vi "worksheet filter column2 lv.vi"(4 "and_or":u8, 6 "lxw_filter_rule 2":T1 {"criteria" items=["LXW_FILTER_CRITERIA_NONE", "LXW_FILTER_CRITERIA_EQUAL_TO", "LXW_FILTER_CRITERIA_NOT_EQUAL_TO", "LXW_FILTER_CRITERIA_GREATER_THAN", "LXW_FILTER_CRITERIA_LESS_THAN", "LXW_FILTER_CRITERIA_GREATER_THAN_OR_EQUAL_TO", "LXW_FILTER_CRITERIA_LESS_THAN_OR_EQUAL_TO", "LXW_FILTER_CRITERIA_BLANKS", "LXW_FILTER_CRITERIA_NON_BLANKS"]}, 8 "error in (no error)":errorcluster, 9 "lxw_filter_rule":T1 {"criteria" items=["LXW_FILTER_CRITERIA_NONE", "LXW_FILTER_CRITERIA_EQUAL_TO", "LXW_FILTER_CRITERIA_NOT_EQUAL_TO", "LXW_FILTER_CRITERIA_GREATER_THAN", "LXW_FILTER_CRITERIA_LESS_THAN", "LXW_FILTER_CRITERIA_GREATER_THAN_OR_EQUAL_TO", "LXW_FILTER_CRITERIA_LESS_THAN_OR_EQUAL_TO", "LXW_FILTER_CRITERIA_BLANKS", "LXW_FILTER_CRITERIA_NON_BLANKS"]}, 10 "col":u16, 11 "worksheet":u32) -> (0 "error out":errorcluster, 3 "function return":u32(ring))   [LabVIEW 8.6]
doc: "lxw_error worksheet_filter_column2(lxw_worksheet worksheet, lxw_col_t col, unsigned long rule1, unsigned long rule2, uint8_t and_or);"
uses:
  pending_lvxlsxwriter/xlsxwriter.dll
  Controls/lxw_filter_criteria.ctl
  Controls/lxw_filter_rule.ctl
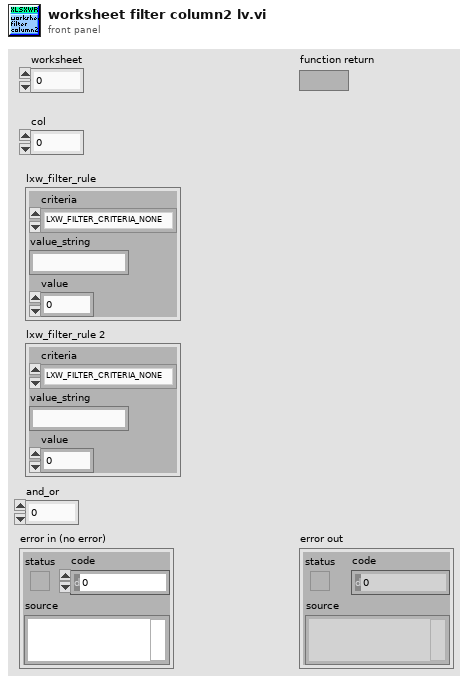
[diagram p1: front panel]
types:
  T1 = typedef "lxw_filter_rule.ctl" = cluster{"criteria":T2, "value_string":string, "value":dbl}
  T2 = typedef "lxw_filter_criteria.ctl" = u32
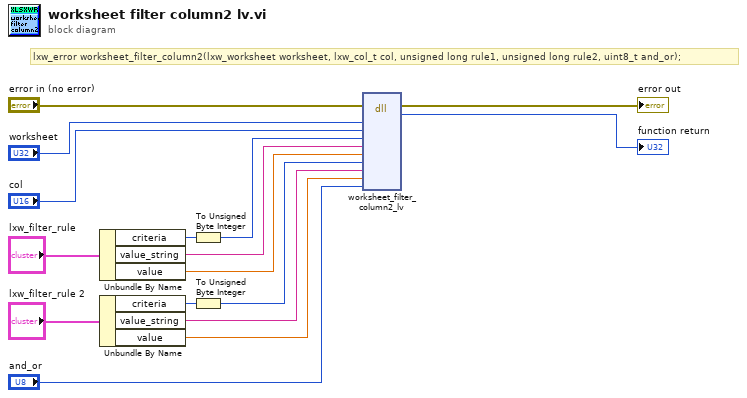
[diagram p0: block diagram]
diagram:
  # "lxw_error worksheet_filter_column2(lxw_worksheet worksheet, lxw_col_t col, unsigned long rule1, unsigned long rule2, uint8_t and_or);"
  n1 = Unbundle By Name("lxw_filter_rule") -> ("criteria"=w11:T2, "value_string"=w8:string, "value"=w7:dbl)
  n2 = Unbundle By Name("lxw_filter_rule 2") -> ("criteria"=w6:T2, "value_string"=w3:string, "value"=w2:dbl)
  n3 = To Unsigned Byte Integer(number=w11) -> (unsigned 8bit integer=w9:u8)
  n4 = To Unsigned Byte Integer(number=w6) -> (unsigned 8bit integer=w4:u8)
  n5 = dll-call lib="C:/Users/WDAGUtilityAccount/Desktop/pending_lvxlsxwriter/xlsxwriter.*" fn="worksheet_filter_column2_lv"(error in="error in (no error)", "worksheet"="worksheet", "col"="col", "criteria1"=w9, "value_string1"=w8, "value1"=w7, "criteria2"=w4, "value_string2"=w3, "value2"=w2, "and_or"="and_or") -> (error out=→"error out":errorcluster, "return type"=→"function return":u32)  [unwired: 11 in, 1 out]
